vi "test.vi"() -> ()   [LabVIEW 2010, in "FPGAWrapperAK101022Resonance.lvclass"]
uses:
  FPGAWrapperAK101022Resonance.lvclass
  scan_specification_cluster.ctl
  class_data.vi
  Program Files/National Instruments/LabVIEW 2010/resource/objmgr/ni.dex.rc
panel:
  out "channelA 2D":dbl[][](graph)
  out "channelA":dbl[](array[numeric])
  out "Available Elements for Reading":i32
  out "DAQ loop error out":errorcluster
  out "FPGA_AK101022Resonance out":refnum<class "FPGAWrapperAK101022Resonance.lvclass">
  in  "scan specification":T1
  in  "number of channels":i32=2
  in  "block size":i32=10000
  out "channel data block":dbl[][](graph)
  in  "timeout (ms)":i32=500
  out "timed out?":bool
  out "DAQ loop counter":i32=9010145
  in  "run button":bool
  in  "stop":bool
  # "Test VI for FGPA_AK101022Resonance"
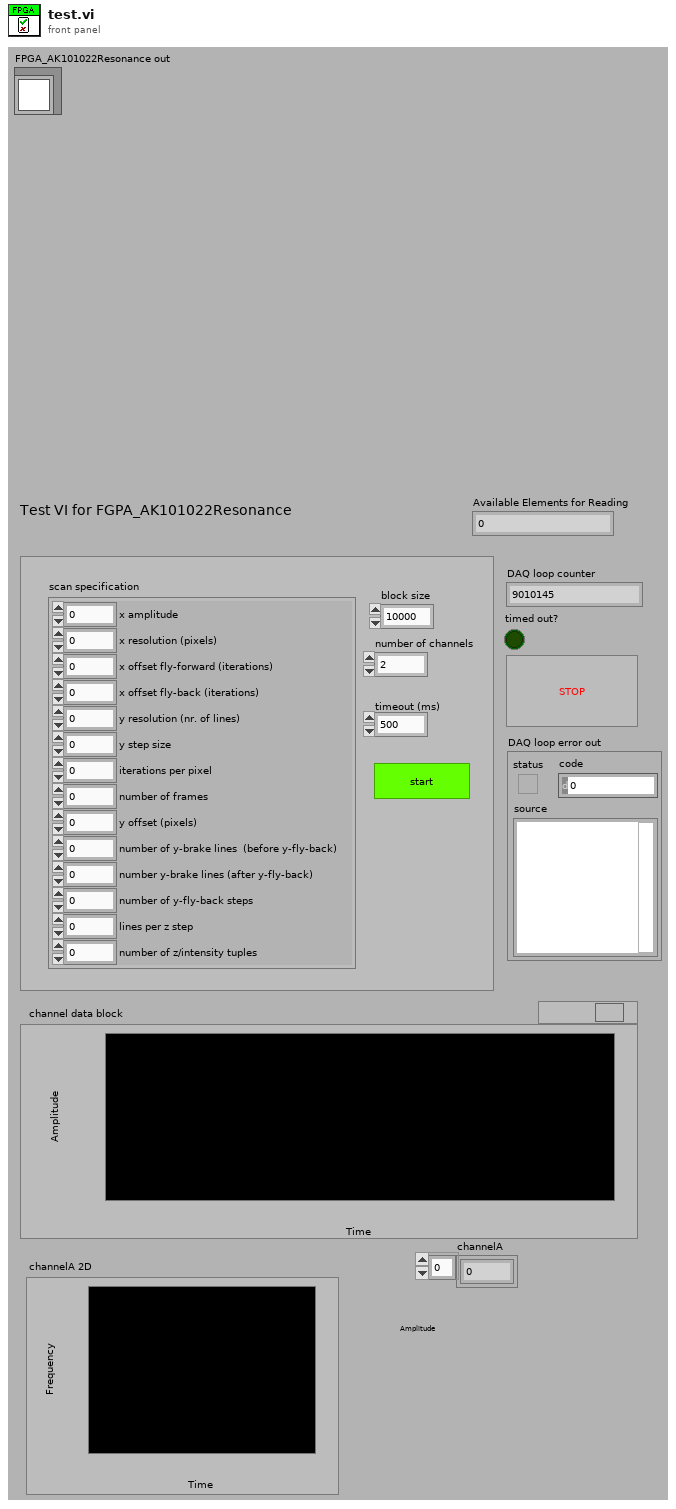
[diagram p1: front panel]
types:
  T1 = typedef "scan_specification_cluster.ctl" = cluster{"x amplitude":u16, "x resolution (pixels)":u16, "x offset fly-forward (iterations)":u16, "x offset fly-back (iterations)":u16, "y resolution (nr. of lines)":u16, "y step size":u16, "iterations per pixel":u16, "number of frames":i32, "y offset (pixels)":u16, "number of y-brake lines  (before y-fly-back)":u16, "number y-brake lines (after y-fly-back)":u16, "number of y-fly-back steps":u16, "lines per z step":u16, "number of z/intensity tuples":u16}
  T2 = typedef "pixel_raw_data_array.ctl" = dbl[][]
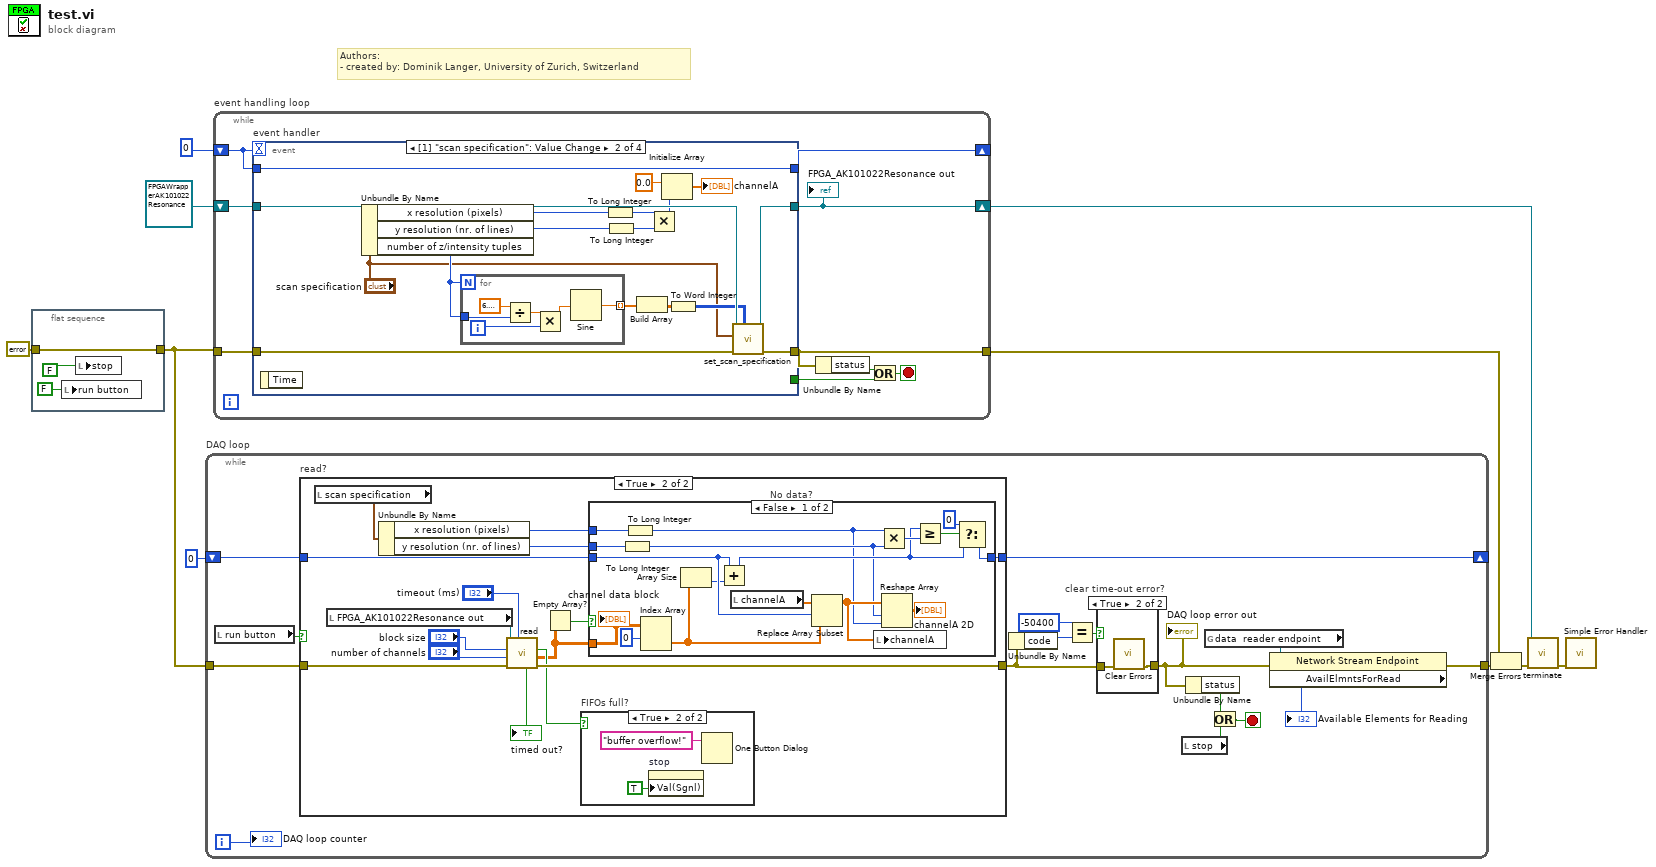
[diagram p0: block diagram]
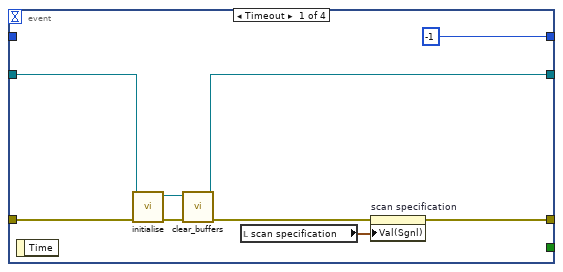
[diagram p6: hidden frame]
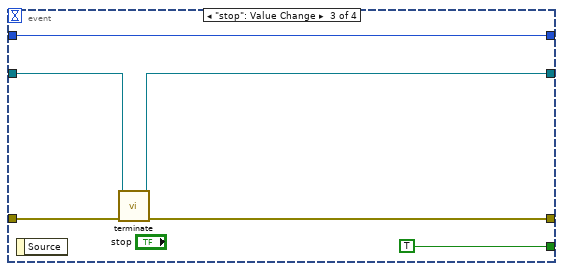
[diagram p7: hidden frame]
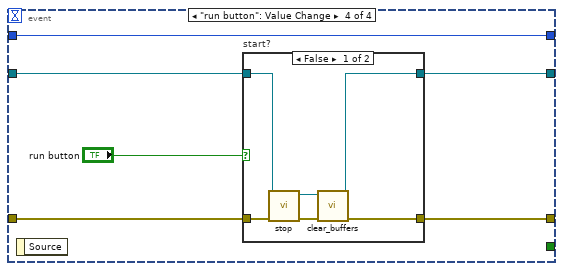
[diagram p8: hidden frame]
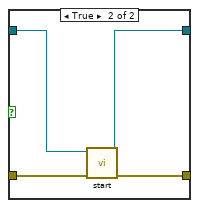
[diagram p9: hidden frame]
diagram:
  # "Authors: \n- created by: Dominik Langer, University of Zurich, Switzerland"
  n1 = flat-sequence {
    tunnel: errorcluster {"status"=FALSE, "code"=0, "source"=""} ("error in (no error)") -> [w13]
    tunnel: [w13] -> w2
    frame #0 {
      n2 = local write "run button"(FALSE ("run button")) -> ()
      n3 = local write "stop"(FALSE) -> ()
    }
  }
  n4 = while "DAQ loop" {
    tunnel: w2 -> [w29]
    tunnel: [w17] -> w9
    shift-right: [w14] -> _
    shift-left: 0 -> [w15]
    i -> [w20]
    stop <- w21 stop-if-true
    n5 = local read "run button"() -> (w28:bool)
    n6 = case "read?" shown="True" w28 {
      tunnel: w29 -> [w33 w48]
      tunnel: [w33 w47] -> w25
      tunnel: w15 -> [_ w38]
      tunnel: [_ w37] -> w14
      frame False {
      }
      frame True {
        n7 = local read "scan specification"() -> (w36:T1)
        n8 = local read "FPGA_AK101022Resonance out"() -> (w41:refnum<class "FPGAWrapperAK101022Resonance.lvclass">)
        n9 = Unbundle By Name(w36) -> ("x resolution (pixels)"=w34:u16, "y resolution (nr. of lines)"=w35:u16)
        n10 = call-dynamic "read.vi"("timeout (ms)"="timeout (ms)", "error in (no error)"=w48, "number of channels"="number of channels", "block size"="block size", "FPGA_AK101022Resonance in"=w41) -> ("error out"=w47:errorcluster, "channels raw data block"=w39:T2, "FIFO full?"=w44:bool, "timed out?"=→"timed out?":bool)  [unwired: 3 out]
        n11 = Empty Array?(array=w39) -> (empty?=w40:bool)
        n12 = case "FIFOs full?" shown="True" w44 {
          frame False {
          }
          frame True {
            n13 = property on="stop" class="Bool (strict)"("Val(Sgnl)"=TRUE) -> ()  [unwired: 2 in, 2 out]
            n14 = One Button Dialog(message="buffer overflow!") -> ()  [unwired: 1 in, 1 out]
          }
        }
        n15 = case "No data?" shown="False" w40 {
          tunnel: w39 -> [w67 _]
          tunnel: w38 -> [w65 w68]
          tunnel: [w58 w68] -> w37
          tunnel: w34 -> [w63 _]
          tunnel: w35 -> [w62 _]
          frame False {
            n16 = To Long Integer(number=w62) -> (32bit integer=w54:i32)
            n17 = To Long Integer(number=w63) -> (32bit integer=w53:i32)
            n18 = Index Array(array=w67, index (row)=0) -> (element=w52:dbl[])  [unwired: 1 in]
            n19 = Array Size(array=w52) -> (size(s)=w51:i32)
            n20 = Add(x=w65, y=w51) -> (x+y=w59:i32)
            n21 = local read "channelA"() -> (w66:dbl[])
            n22 = Replace Array Subset(array=w66, new element=w52, index=w65) -> (w55:dbl[])
            n23 = local write "channelA"(w55) -> ()
            n24 = Multiply(x=w53, y=w54) -> (x*y=w61:i32)
            n25 = Reshape Array(w55, w54, w53) -> (→"channelA 2D":dbl[][])
            n26 = Greater Or Equal?(x=w59, y=w61) -> (x >= y?=w60:bool)
            n27 = Select(t=0, s=w60, f=w59) -> (s? t:f=w58:i32)
            "channel data block" <- w67
          }
          frame True {
          }
        }
      }
    }
    n28 = Unbundle By Name(w25) -> ("code"=w27:i32)
    n29 = Equal?(x=-50400, y=w27) -> (x = y?=w24:bool)
    n30 = case "clear time-out error?" shown="True" w24 {
      tunnel: w25 -> [w30 w32]
      tunnel: [w30 w31] -> w18
      frame False {
      }
      frame True {
        n31 = call <vilib>:"Clear Errors.vi"("error in (no error)"=w32) -> ("error out"=w31:errorcluster)  [unwired: 6 out]
      }
    }
    "DAQ loop error out" <- w18
    n32 = local read "stop"() -> (w22:bool)
    n33 = Unbundle By Name(w18) -> ("status"=w23:bool)
    n34 = global read "class_data.vi" "data  reader endpoint"() -> (w19:refnum<k21>)
    n35 = Or(x=w23, y=w22) -> (x .or. y?=w21:bool)
    n36 = property class="Network Stream Endpoint"(reference=w19, error in=w18) -> (error out=w17:errorcluster, "AvailElmntsForRead"=→"Available Elements for Reading":i32)  [unwired: 1 out]
    "DAQ loop counter" <- w20
  }
  n37 = while "event handling loop" {
    shift-right: [w75] -> _
    shift-left: 0 -> [w76]
    shift-right: [w73] -> w8
    shift-left: refnum<class "FPGAWrapperAK101022Resonance.lvclass"> refnum ("FPGA_AK101022Resonance.lvclass") -> [w74]
    tunnel: w2 -> [w77]
    tunnel: [w72] -> w7
    stop <- w69 stop-if-true
    n38 = event "event handler" shown="[1] \"scan specification\": Value Change" {
      selector: _ -> [_ _ _ _]
      dyn-events: _ -> [_ _ _ _]
      timeout: w76 -> [_ _ _ _]
      tunnel: [w83 w99 w112 w116] -> w72
      tunnel: w77 -> [w84 w100 w113 w120]
      tunnel: w76 -> [_ w103 w115 w121]
      tunnel: [-1 w103 w115 w121] -> w75
      tunnel: [_ _ TRUE _] -> w70
      tunnel: [w79 w101 w110 w117] -> w73
      tunnel: w74 -> [w85 w102 w111 w118]
      event Timeout {
        n39 = event-data() -> ()  [unwired: 2 out]
        n40 = call-dynamic "initialise.vi"("error in (no error)"=w84, "FPGA_AK101022Resonance in"=w85) -> ("error out"=w82:errorcluster, "FPGA_AK101022Resonance out"=w80:refnum<class "FPGAWrapperAK101022Resonance.lvclass">)  [unwired: 8 in]
        n41 = call-dynamic "clear_buffers.vi"("error in (no error)"=w82, "FPGA_AK101022Resonance in"=w80) -> ("error out"=w81:errorcluster, "FPGA_AK101022Resonance out"=w79:refnum<class "FPGAWrapperAK101022Resonance.lvclass">)  [unwired: 8 in]
        n42 = local read "scan specification"() -> (w78:T1)
        n43 = property on="scan specification" class="Clust (strict)"(error in=w81, "Val(Sgnl)"=w78) -> (error out=w83:errorcluster)  [unwired: 1 in, 1 out]
      }
      event Value Change {
        n44 = event-data() -> ()  [unwired: 2 out]
        n45 = Unbundle By Name("scan specification") -> ("x resolution (pixels)"=w97:u16, "y resolution (nr. of lines)"=w93:u16, "number of z/intensity tuples"=w91:u16)
        n46 = for {
          N: w91 -> [_]
          tunnel: w91 -> [w108]
          tunnel: [w104] -> w90 mode=indexing
          i -> [w106]
          n47 = Divide(x=6.283185307179586, y=w108) -> (x/y=w107:dbl)
          n48 = Multiply(x=w107, y=w106) -> (x*y=w105:dbl)
          n49 = Sine(x=w105) -> (sin(x)=w104:dbl)
        }
        n50 = To Long Integer(number=w97) -> (32bit integer=w94:i32)
        n51 = To Long Integer(number=w93) -> (32bit integer=w92:i32)
        n52 = Build Array(w90, w90) -> (w89:dbl[][])
        n53 = Multiply(x=w94, y=w92) -> (x*y=w95:i32)
        n54 = Initialize Array(0.0 ("element"), w95) -> (→"channelA":dbl[])
        n55 = To Word Integer(number=w89) -> (16bit integer=w88:i16[][])
        n56 = call-dynamic "set_scan_specification.vi"("z/intensity tuples (1st row: z values, 2nd row intensity values)"=w88, "error in (no error)"=w100, "scan specification"="scan specification", "FPGA_AK101022Resonance in"=w102) -> ("error out"=w99:errorcluster, "FPGA_AK101022Resonance out"=w101:refnum<class "FPGAWrapperAK101022Resonance.lvclass">)  [unwired: 6 in]
      }
      event "stop": Value Change {
        n57 = event-data() -> ()  [unwired: 2 out]
        n58 = call-dynamic "terminate.vi"("error in (no error)"=w113, "FPGA_AK101022Resonance in"=w111) -> ("error out"=w112:errorcluster, "FPGA_AK101022Resonance out"=w110:refnum<class "FPGAWrapperAK101022Resonance.lvclass">)  [unwired: 8 in]
      }
      event "run button": Value Change {
        n59 = event-data() -> ()  [unwired: 2 out]
        n60 = case "start?" shown="False" "run button" {
          tunnel: w120 -> [w127 w129]
          tunnel: w118 -> [w126 w128]
          tunnel: [w122 w131] -> w117
          tunnel: [w124 w130] -> w116
          frame False {
            n61 = call-dynamic "stop.vi"("error in (no error)"=w127, "FPGA_AK101022Resonance in"=w126) -> ("error out"=w125:errorcluster, "FPGA_AK101022Resonance out"=w123:refnum<class "FPGAWrapperAK101022Resonance.lvclass">)  [unwired: 8 out]
            n62 = call-dynamic "clear_buffers.vi"("error in (no error)"=w125, "FPGA_AK101022Resonance in"=w123) -> ("error out"=w124:errorcluster, "FPGA_AK101022Resonance out"=w122:refnum<class "FPGAWrapperAK101022Resonance.lvclass">)  [unwired: 8 in]
          }
          frame True {
            n63 = call-dynamic "start.vi"("error in (no error)"=w129, "FPGA_AK101022Resonance in"=w128) -> ("error out"=w130:errorcluster, "FPGA_AK101022Resonance out"=w131:refnum<class "FPGAWrapperAK101022Resonance.lvclass">)  [unwired: 8 out]
          }
        }
      }
    }
    "FPGA_AK101022Resonance out" <- w73
    n64 = Unbundle By Name(w72) -> ("status"=w71:bool)
    n65 = Or(x=w71, y=w70) -> (x .or. y?=w69:bool)
  }
  n66 = call-dynamic "terminate.vi"("error in (no error)"=w9, "FPGA_AK101022Resonance in"=w8) -> ("error out"=w6:errorcluster)  [unwired: 9 out]
  n67 = Merge Errors(w7, w6) -> (w5:errorcluster)
  n68 = call <vilib>:"Simple Error Handler.vi"("error in (no error)"=w5) -> ()  [unwired: 1 in, 8 out]
